vi "Single Tone Measurement (IO).vi"(8 "error in (no error)":errorcluster, 10 "sweep start frequency (Hz)":dbl, 11 "measurement configuration":T2 {"acq sampling rate" format="%0.2f"; "master clock rate" format="%#_6pHz"; "frame clock rate" format="%#_6pHz"}) -> (0 "error out":errorcluster, 1 "spectrum":cluster{"x0":dbl, "dx":dbl, "magnitude":dbl[]}, 2 "time domain":waveform(dbl), 3 "results":T1, 4 "output power":dbl)   [LabVIEW 2021, in "Stepped Frequency Sweep_Class D Amplifier.lvlib"]
uses:
  Measurement Configuration.ctl
  shared/controls/digital audio protocol/data justification.ctl
  shared/controls/digital audio protocol/endianness.ctl
  shared/controls/digital audio protocol/digital edge.ctl
  shared/controls/digital audio protocol/logic level.ctl
  shared/controls/digital output level units.ctl
  shared/controls/weighting filter.ctl
  shared/controls/highpass filter.ctl
  shared/controls/lowpass filter.ctl
  shared/controls/sweep profile.ctl
  shared/controls/units - snr.ctl
  shared/controls/units - ratio.ctl
  shared/controls/regulation target.ctl
  shared/controls/single tone audio measurements.ctl
  <vilib>/PDM Acquisition Toolkit/shared/controls/clock mode.ctl
  <vilib>/PDM Acquisition Toolkit/shared/controls/PCM Frame Sync Control.ctl
  <vilib>/PDM Acquisition Toolkit/shared/controls/Digital Edge.ctl
  <vilib>/PDM Acquisition Toolkit/shared/controls/PCM Data Format Configuration.ctl
  <vilib>/PDM Acquisition Toolkit/shared/controls/PCM Bit Endianness.ctl
  <vilib>/PDM Acquisition Toolkit/shared/controls/PCM Data Justification.ctl
  shared/controls/single tone audio measurement settings.ctl
  shared/controls/audio filter settings.ctl
  shared/controls/units settings.ctl
  <vilib>/DAQmx/read.llb/DAQmx Read (Analog 1D Wfm NChan NSamp).vi
  <vilib>/DAQmx/create/channels.llb/DAQmx Create Channel (AI-Voltage-Basic).vi
  <vilib>/DAQmx/configure/timing.llb/DAQmx Timing (Sample Clock).vi
  <vilib>/PDM Acquisition Toolkit/host/API/Public/Function Generator/Configure Custom Signal (N Ch) - PCM Output Task.vi
  <vilib>/DAQmx/miscellaneous.llb/DAQmx Fill In Error Info.vi
  <vilib>/Waveform/WDTOps.llb/WDT Get Waveform Subset DBL.vi
  Stepped Frequency Sweep_Class D Amplifier.lvlib
  <vilib>/PDM Acquisition Toolkit/shared/PDM Shared.lvlib
  <vilib>/PDM Acquisition Toolkit/host/API/PDM Acquisition Toolkit.lvlib
  shared/controls/audio controls.lvlib
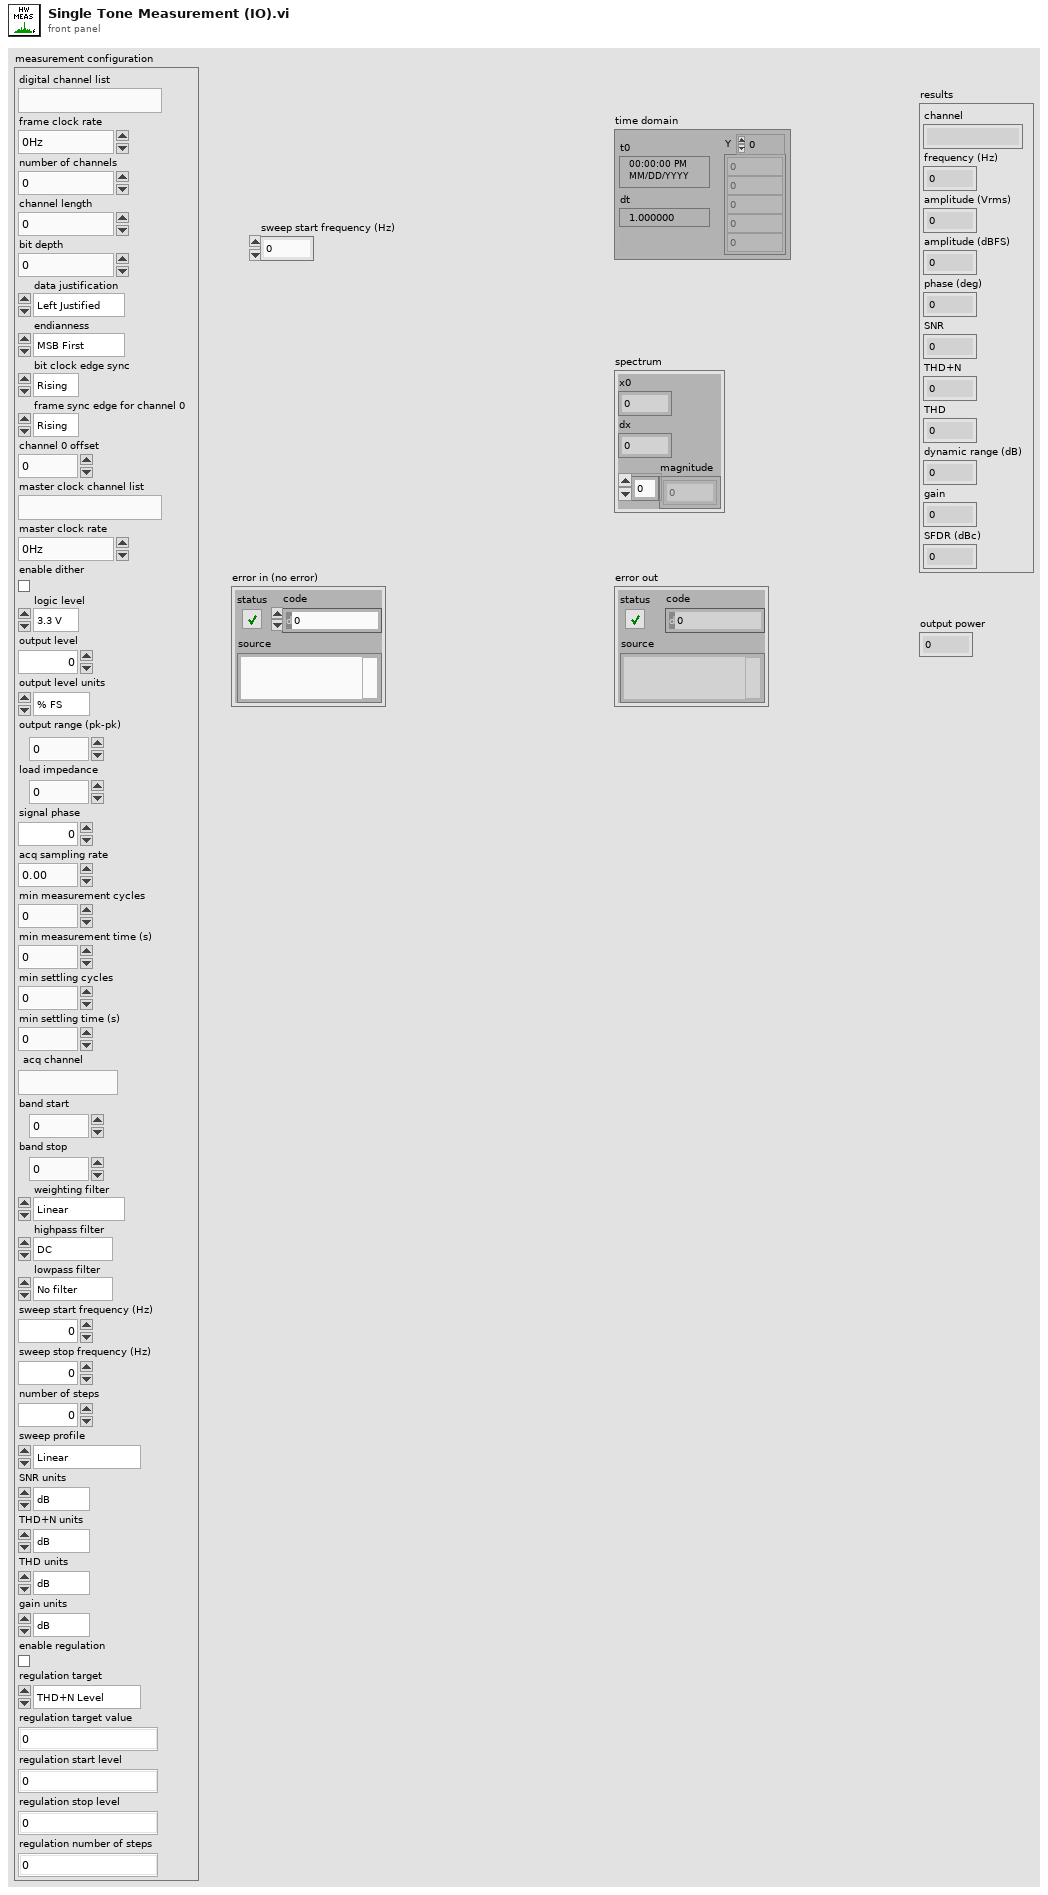
[diagram p1: front panel]
types:
  T1 = typedef "audio controls.lvlib/single tone audio measurements.ctl" = cluster{"channel":string, "frequency (Hz)":dbl, "amplitude (Vrms)":dbl, "amplitude (dBFS)":dbl, "phase (deg)":dbl, "SNR":dbl, "THD+N":dbl, "THD":dbl, "dynamic range (dB)":dbl, "gain":dbl, "SFDR (dBc)":dbl}
  T2 = typedef "Stepped Frequency Sweep_Class D Amplifier.lvlib/Measurement Configuration.ctl" = cluster{"digital channel list":string, "frame clock rate":dbl, "number of channels":u32, "channel length":u32, "bit depth":u32, "data justification":T3, "endianness":T4, "bit clock edge sync":T5, "frame sync edge for channel 0":T5, "channel 0 offset":u32, "master clock channel list":string, "master clock rate":dbl, "enable dither":bool, "logic level":T6, "output level":dbl, "output level units":T7, "output range (pk-pk)":dbl, "load impedance":dbl, "signal phase":dbl, "acq sampling rate":dbl, "min measurement cycles":u32, "min measurement time (s)":dbl, "min settling cycles":u32, "min settling time (s)":dbl, "acq channel":string, "band start":dbl, "band stop":dbl, "weighting filter":T8, "highpass filter":T9, "lowpass filter":T10, "sweep start frequency (Hz)":dbl, "sweep stop frequency (Hz)":dbl, "number of steps":u32, "sweep profile":T11, "SNR units":T12, "THD+N units":T13, "THD units":T13, "gain units":T13, "enable regulation":bool, "regulation target":T14, "regulation target value":dbl, "regulation start level":dbl, "regulation stop level":dbl, "regulation number of steps":u32}
  T3 = typedef "data justification.ctl" = enum32{"Left Justified", "Right Justified"}
  T4 = typedef "endianness.ctl" = enum32{"MSB First", "LSB First"}
  T5 = typedef "digital edge.ctl" = enum32{"Rising", "Falling"}
  T6 = typedef "logic level.ctl" = enum32{"3.3 V", "1.8 V", "1.2 V"}
  T7 = typedef "audio controls.lvlib/digital output level units.ctl" = enum32{"% FS", "dBFS"}
  T8 = typedef "weighting filter.ctl" = enum32{"Linear", "A-weighting", "B-weighting", "C-weighting"}
  T9 = typedef "highpass filter.ctl" = enum32{"DC", "AC"}
  T10 = typedef "lowpass filter.ctl" = enum32{"No filter", "AES17 20kHz", "AES17 40kHz"}
  T11 = typedef "audio controls.lvlib/sweep profile.ctl" = enum32{"Linear", "Logarithmic"}
  T12 = typedef "audio controls.lvlib/units - snr.ctl" = enum32{"dB", "x/y"}
  T13 = typedef "audio controls.lvlib/units - ratio.ctl" = enum32{"dB", "%", "x/y"}
  T14 = typedef "regulation target.ctl" = enum32{"THD+N Level", "THD+N Ratio", "RMS Level", "RMS Ratio", "Output Power"}
  T15 = typedef "audio controls.lvlib/units settings.ctl" = cluster{"SNR units":T12, "THD+N units":T13, "THD units":T13, "gain units":T13}
  T16 = typedef "audio filter settings.ctl" = cluster{"weighting filter":T8, "highpass filter":T9, "lowpass filter ":T10}
  T17 = typedef "single tone audio measurement settings.ctl" = cluster{"Band start":dbl, "Band stop":dbl, "Amplitude":dbl, "Frequency":dbl, "Full scale range":dbl}
  T18 = typedef "PDM Shared.lvlib/PCM Data Format Configuration.ctl" = cluster{"Frame Sync Edge for Channel 0":T19, "Channel Count Per Frame":u8, "Channel Length":u16, "Bit Depth":u8, "Channel 0 Offset":u16, "Endianness":T20, "Data Justification":T21}
  T19 = typedef "PDM Shared.lvlib/Digital Edge.ctl" = enum8{"Rising", "Falling"}
  T20 = typedef "PDM Shared.lvlib/PCM Bit Endianness.ctl" = enum16{"MSB First", "LSB First"}
  T21 = typedef "PDM Shared.lvlib/PCM Data Justification.ctl" = enum16{"Left Justified", "Right Justified"}
  T22 = typedef "PDM Shared.lvlib/PCM Frame Sync Control.ctl" = cluster{"Frame Length":u16, "Frame Sync Pulse Width":u16, "Bit Clock Edge  Sync":T19}
  T23 = typedef "PDM Shared.lvlib/clock mode.ctl" = enum16{"divided clock", "DDS"}
  T24 = typedef "PDM Acquisition Class Library.lvlib/PCM Output Task.lvclass/PCM Output Task DVR.ctl" = refnum<data-value>
  T25 = typedef "PDM Acquisition Class Library.lvlib/I2S Output Task.lvclass/SignalProperties.ctl" = cluster{"cyclic signal":dbl[], "channel parameters":T26[]}
  T26 = typedef "PDM Acquisition Class Library.lvlib/I2S Output Channel.lvclass/GenerationChannelProperties.ctl" = cluster{"cyclic period":dbl, "cyclic phase offset":dbl, "gain":dbl}
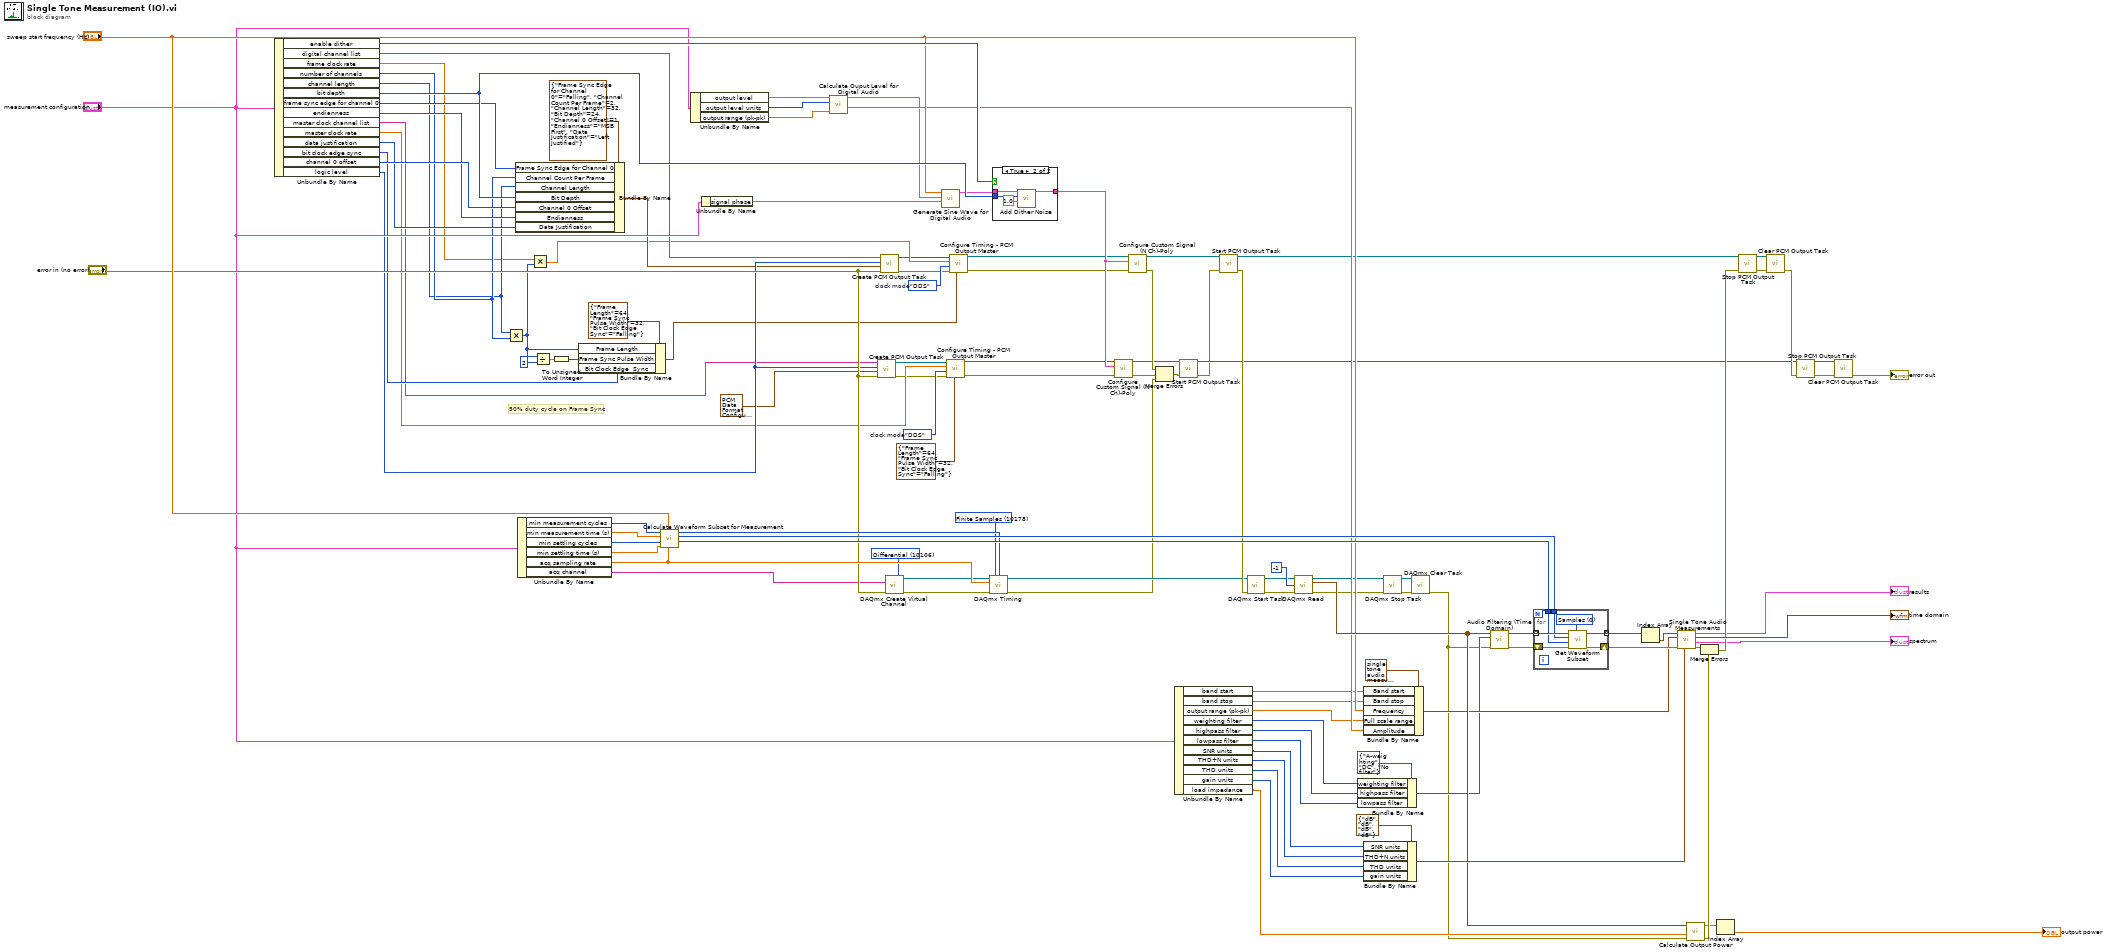
[diagram p0: block diagram]
diagram:
  w56 = 10106 items=["Default"=-1, "RSE"=10083, "NRSE"=10078, "Differential"=10106, "Pseudodifferential"=12529] ("input terminal configuration")
  w43 = 10178 items=["Finite Samples"=10178, "Continuous Samples"=10123, "Hardware Timed Single Point"=12522] ("sample mode")
  w8 = clock_mode."DDS"  # clock mode
  w5 = clock_mode."DDS"  # clock mode
  # "50% duty cycle on Frame Sync"
  n1 = Unbundle By Name("measurement configuration") -> ("enable dither"=w114:bool, "digital channel list"=w70:string, "frame clock rate"=w47:dbl, "number of channels"=w49:u32, "channel length"=w48:u32, "bit depth"=w113:u32, "frame sync edge for channel 0"=w59:T5, "endianness"=w60:T4, "master clock channel list"=w50:string, "master clock rate"=w51:dbl, "data justification"=w58:T3, "bit clock edge sync"=w61:T5, "channel 0 offset"=w62:u32, "logic level"=w63:T6)
  n2 = Multiply(x=w48, y=w49) -> (x*y=w22:u32)
  n3 = Bundle By Name(cluster=T18 {"Frame Sync Edge for Channel 0"=enum."Falling", "Channel Count Per Frame"=2, "Channel Length"=32, "Bit Depth"=24, "Channel 0 Offset"=1, "Endianness"=enum."MSB First", "Data Justification"=enum."Left Justified"} ("PCM Data Configuration"), "Frame Sync Edge for Channel 0"=w59, "Channel Count Per Frame"=w49, "Channel Length"=w48, "Bit Depth"=w113, "Channel 0 Offset"=w62, "Endianness"=w60, "Data Justification"=w58) -> (w25:T18)
  n4 = Unbundle By Name("measurement configuration") -> ("min measurement cycles"=w100:u32, "min measurement time (s)"=w101:dbl, "min settling cycles"=w102:u32, "min settling time (s)"=w103:dbl, "acq sampling rate"=w91:dbl, "acq channel"=w55:string)
  n5 = Multiply(x=w47, y=w22) -> (x*y=w23:dbl)
  n6 = Divide(x=w22, y=u16 2) -> (x/y=w20:dbl)
  n7 = To Unsigned Word Integer(number=w20) -> (unsigned 16bit integer=w21:u16)
  n8 = Bundle By Name(cluster=T22 {"Frame Length"=64, "Frame Sync Pulse Width"=32, "Bit Clock Edge  Sync"=enum."Falling"} ("Frame Sync Clock Control"), "Frame Length"=w22, "Frame Sync Pulse Width"=w21, "Bit Clock Edge  Sync"=w61) -> (w18:T22)
  n9 = call "Calculate Waveform Subset for Measurement.vi"("sampling rate"=w91, "signal frequency"="sweep start frequency (Hz)", "minimum settling duration"=w103, "minimum settling cycles"=w102, "minimum measurement duration"=w101, "minimum measurement cycles"=w100) -> ("duration (samples)"=w99:u32, "start (samples)"=w98:u32, "total acquisition (samples)"=w92:u32)  [unwired: 3 in]
  n10 = Unbundle By Name("measurement configuration") -> ("output level"=w74:dbl, "output level units"=w75:T7, "output range (pk-pk)"=w76:dbl)
  n11 = Unbundle By Name("measurement configuration") -> ("signal phase"=w64:dbl)
  n12 = call "Calculate Ouput Level for Digital Audio.vi"("output range (pk-pk)"=w76, "digital output level units"=w75, "output level"=w74) -> ("amplitude (pk)"=w77:dbl, "gain"=w71:dbl)  [unwired: 7 in]
  n13 = call <vilib>:"Create PCM Output Task.vi"("error in"="error in (no error)", "PCM data configuration"=T18 {"Frame Sync Edge for Channel 0"=enum."Falling", "Channel Count Per Frame"=2, "Channel Length"=32, "Bit Depth"=24, "Channel 0 Offset"=1, "Endianness"=enum."MSB First", "Data Justification"=enum."Left Justified"} ("PCM Data Configuration 2"), "logic level"=w63, "channel list"=w50) -> ("error out"=w7:errorcluster, "PCM output task out"=w6:T24)  [unwired: 6 in]
  n14 = call <vilib>:"Create PCM Output Task.vi"("error in"="error in (no error)", "PCM data configuration"=w25, "logic level"=w63, "channel list"=w70) -> ("error out"=w4:errorcluster, "PCM output task out"=w3:T24)  [unwired: 6 in]
  n15 = call-poly <vilib>:"DAQmx Create Virtual Channel.vi"("input terminal configuration"=w56, "physical channels"=w55, "error in"="error in (no error)") -> ("task out"=w34:refnum<k21>, "error out"=w33:errorcluster)  [unwired: 11 in]
  n16 = call "Generate Sine Wave for Digital Audio.vi"("phase"=w64, "gain"=w71, "frequency"="sweep start frequency (Hz)") -> ("Signal Properties"=w111:T25)  [unwired: 8 in]
  n17 = call <vilib>:"Configure Timing - PCM Output Master.vi"("Frame Sync Clock Control"=T22 {"Frame Length"=64, "Frame Sync Pulse Width"=32, "Bit Clock Edge  Sync"=enum."Falling"} ("Frame Sync Clock Control 2"), "error in"=w7, "clock mode"=w8, "Bit Clock rate"=w51, "PCM output task in"=w6) -> ("error out"=w26:errorcluster, "PCM output task out"=w27:T24)  [unwired: 4 in, 1 out]
  n18 = call <vilib>:"Configure Timing - PCM Output Master.vi"("Frame Sync Clock Control"=w18, "error in"=w4, "clock mode"=w5, "Bit Clock rate"=w23, "PCM output task in"=w3) -> ("error out"=w73:errorcluster, "PCM output task out"=w72:T24)  [unwired: 4 in, 1 out]
  n19 = call-poly <vilib>:"DAQmx Timing.vi"("task/channels in"=w34, "sample mode"=w43, "samples per channel"=w92, "rate"=w91, "error in"=w33) -> ("task out"=w42:refnum<k21>, "error out"=w41:errorcluster)  [unwired: 9 in]
  n20 = case shown="True" w114 {
    tunnel: w111 -> [w116 w120]
    tunnel: [w116 w119] -> w112
    tunnel: w113 -> [_ w118]
    frame False {
    }
    frame True {
      n21 = call "Add Dither Noise.vi"("amplitude (LSB)"=1.0, "bits"=w118, "Signal Properties"=w120) -> ("Signal Properties"=w119:T25)  [unwired: 8 in]
    }
  }
  n22 = call-poly <vilib>:"Configure Custom Signal (N Ch)-Poly.vi"("error in"=w26, "signal parameters"=w112, "PCM output task in"=w27) -> ("error out"=w31:errorcluster, "PCM output task out"=w28:T24)  [unwired: 7 in]
  n23 = call-poly <vilib>:"Configure Custom Signal (N Ch)-Poly.vi"("error in"=w73, "signal parameters"=w112, "PCM output task in"=w72) -> ("error out"=w30:errorcluster, "PCM output task out"=w29:T24)  [unwired: 7 in]
  n24 = Merge Errors(w30, w31, w41) -> (w12:errorcluster)
  n25 = Unbundle By Name("measurement configuration") -> ("band start"=w53:dbl, "band stop"=w54:dbl, "output range (pk-pk)"=w69:dbl, "weighting filter"=w86:T8, "highpass filter"=w87:T9, "lowpass filter"=w88:T10, "SNR units"=w106:T12, "THD+N units"=w107:T13, "THD units"=w108:T13, "gain units"=w109:T13, "load impedance"=w110:dbl)
  n26 = call <vilib>:"Start PCM Output Task.vi"("error in"=w12, "PCM output task in"=w28) -> ("error out"=w11:errorcluster, "PCM output task out"=w15:T24)  [unwired: 8 in]
  n27 = call <vilib>:"Start PCM Output Task.vi"("error in"=w11, "PCM output task in"=w29) -> ("error out"=w57:errorcluster, "PCM output task out"=w32:T24)  [unwired: 8 in]
  n28 = call <vilib>:"DAQmx Start Task.vi"("task/channels in"=w42, "error in"=w57) -> ("task out"=w39:refnum<k21>, "error out"=w36:errorcluster)  [unwired: 12 in]
  n29 = call-poly <vilib>:"DAQmx Read.vi"("task/channels in"=w39, "number of samples per channel"=-1, "error in"=w36) -> ("task out"=w40:refnum<k21>, "data"=w93:waveform(dbl)[], "error out"=w37:errorcluster)  [unwired: 10 in]
  n30 = Bundle By Name(cluster=T16 {"weighting filter"=enum."A-weighting", "highpass filter"=enum."DC", "lowpass filter "=enum."No filter"} ("filter settings"), "weighting filter"=w86, "highpass filter"=w87, "lowpass filter"=w88) -> (w84:T16)
  n31 = Bundle By Name(cluster=T17 {"Band start"=20.0, "Band stop"=20000.0, "Amplitude"=-1.0, "Frequency"=1000.0, "Full scale range"=15.0} ("measurement settings"), "Band start"=w53, "Band stop"=w54, "Frequency"="sweep start frequency (Hz)", "Full scale range"=w69, "Amplitude"=w77) -> (w85:T17)
  n32 = Bundle By Name(cluster=T15 {"SNR units"=enum."dB", "THD+N units"=enum."dB", "THD units"=enum."dB", "gain units"=enum."dB"} ("units settings"), "SNR units"=w106, "THD+N units"=w107, "THD units"=w108, "gain units"=w109) -> (w105:T15)
  n33 = call <vilib>:"DAQmx Stop Task.vi"("task/channels in"=w40, "error in"=w37) -> ("task out"=w35:refnum<k21>, "error out"=w38:errorcluster)  [unwired: 12 in]
  n34 = call <vilib>:"DAQmx Clear Task.vi"("task in"=w35, "error in"=w38) -> ("error out"=w82:errorcluster)  [unwired: 13 in]
  n35 = call "Audio Filtering (Time Domain).vi"("waveforms"=w93, "filter settings"=w84, "error in"=w82) -> ("time domain"=w95:waveform(dbl)[], "error out"=w94:errorcluster)  [unwired: 6 in]
  n36 = for {
    tunnel: w95 -> [w127] mode=indexing
    tunnel: [w126] -> w96 mode=indexing
    shift-right: [w123] -> w97
    shift-left: w94 -> [w124]
    tunnel: w98 -> [w122]
    tunnel: w99 -> [w121]
    w125 = u16 0 items=["Samples", "Relative Time"] ("start/duration format")
    n37 = call-poly <vilib>:"Get Waveform Subset.vi"("start/duration format"=w125, "error in (no error)"=w124, "duration"=w121, "start samples/time"=w122, "waveform in"=w127) -> ("error out"=w123:errorcluster, "waveform out"=w126:waveform(dbl))  [unwired: 1 in, 2 out]
  }
  n38 = Index Array(array=w96) -> (element=w89:waveform(dbl))  [unwired: 1 in]
  n39 = call "Single Tone Audio Measurements.vi"("units settings"=w105, "error in"=w97, "measurement settings"=w85, "waveform"=w89) -> ("error out"=w66:errorcluster, "spectrum"=→"spectrum":cluster{"x0":dbl, "dx":dbl, "magnitude":dbl[]}, "time domain"=→"time domain":waveform(dbl), "results"=→"results":T1)  [unwired: 4 in]
  n40 = call "Calculate Output Power.vi"("error in (no error)"=w82, "load impedance"=w110, "waveforms"=w93) -> ("error out"=w68:errorcluster, "output power"=w65:dbl[])  [unwired: 7 in]
  n41 = Merge Errors(w66, w68) -> (w67:errorcluster)
  n42 = Index Array(array=w65) -> (element=→"output power":dbl)  [unwired: 1 in]
  n43 = call <vilib>:"Stop PCM Output Task.vi"("error in"=w67, "PCM output task In"=w32) -> ("error out"=w1:errorcluster, "PCM output task out"=w2:T24)  [unwired: 8 in]
  n44 = call <vilib>:"Clear PCM Output Task.vi"("error in"=w1, "PCM output task in"=w2) -> ("error out"=w16:errorcluster)  [unwired: 9 in]
  n45 = call <vilib>:"Stop PCM Output Task.vi"("error in"=w16, "PCM output task In"=w15) -> ("error out"=w13:errorcluster, "PCM output task out"=w14:T24)  [unwired: 8 in]
  n46 = call <vilib>:"Clear PCM Output Task.vi"("error in"=w13, "PCM output task in"=w14) -> ("error out"=→"error out":errorcluster)  [unwired: 9 in]
